vi "Parse Array Data.vi"(0 "Samples String":string, 5 "Current Index":i32=1, 7 "Number of Samples":u32, 11 "error in (no error)":errorcluster) -> (4 "Samples":dbl[](array[numeric]), 6 "Next Index":i32=1, 10 "Stop Reading Samples":bool, 15 "error out":errorcluster)   [LabVIEW 2020]
doc: "Converts the read samples to a double array and checks to see if all samples have been read yet. Also computes the next index to read remaining samples from the Instrument capture buffer."
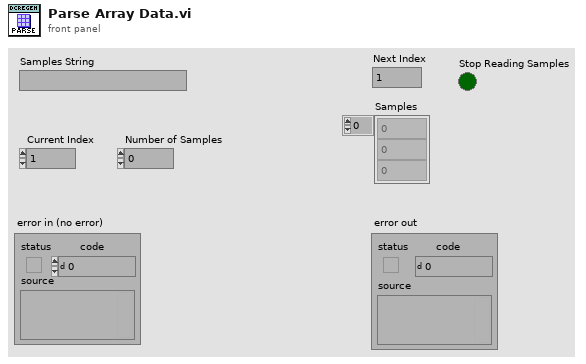
[diagram p1: front panel]
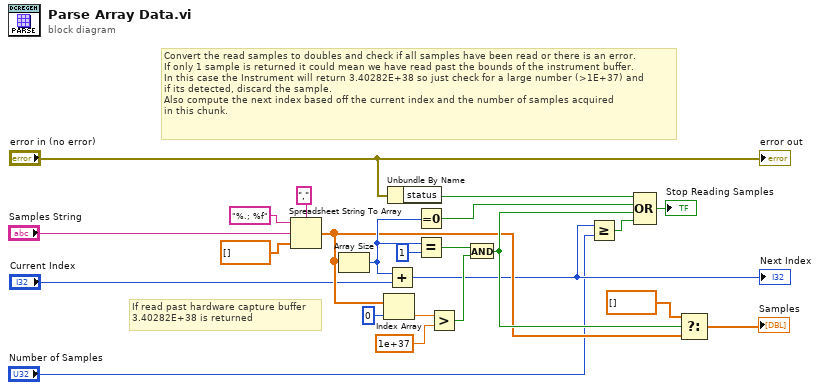
[diagram p0: block diagram]
diagram:
  # "Convert the read samples to doubles and check if all samples have been read or there is an error.\nIf only 1 sample is returned it could mean we have read past the bounds of the instrument buffer.\nIn this case the Instrument will return 3.40282E+38 so just check for a large number (>1E+37) and\nif its detected, discard the sample.\nAlso compute the next index based off the current index and the number of samples acquired\nin this chunk."
  # "If read past hardware capture buffer\n3.40282E+38 is returned"
  n1 = Spreadsheet String To Array(delimiter (Tab)=",", format string="%.; %f", spreadsheet string="Samples String", array type (2D Dbl)=dbl[] []) -> (array=w9:dbl[])
  n2 = Array Size(array=w9) -> (size(s)=w18:i32)
  n3 = Index Array(array=w9, index=0) -> (element=w14:dbl)
  n4 = Add(x=w18, y="Current Index") -> (x+y=w5:i32)
  "Next Index" <- w5
  n5 = Unbundle By Name("error in (no error)") -> ("status"=w20:bool)
  n6 = Equal To 0?(x=w18) -> (x = 0?=w11:bool)
  n7 = Equal?(x=w18, y=1) -> (x = y?=w16:bool)
  n8 = Greater?(x=w14, y=1e+37) -> (0:w12:bool)
  n9 = And(x=w16, y=w12) -> (x .and. y?=w10:bool)
  n10 = Greater Or Equal?(x=w5, y="Number of Samples") -> (x >= y?=w19:bool)
  n11 = Compound Arithmetic op=OR(w20, w11, w10, w19) -> (→"Stop Reading Samples":bool)
  n12 = Select(t=dbl[] [] ("array"), s=w10, f=w9) -> (s? t:f=→"Samples":dbl[])
  "error out" <- "error in (no error)"
